vi "ConvertTemperatureToVoltage.vi"(1 "Température\nde consigne":dbl) -> (0 "Numérique":dbl)   [LabVIEW 2021]
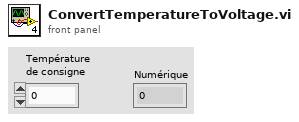
[diagram p1: front panel]
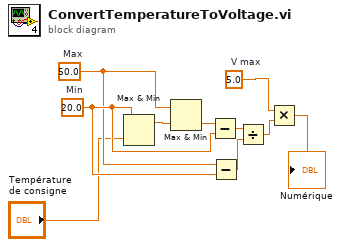
[diagram p0: block diagram]
diagram:
  w9 = 5.0  # V max
  w4 = 50.0  # Max
  w5 = 20.0  # Min
  n1 = Max & Min(x=w5, y="Température\nde consigne") -> (max(x,y)=w2:dbl)  [unwired: 1 out]
  n2 = Max & Min(x=w4, y=w2) -> (min(x,y)=w3:dbl)  [unwired: 1 out]
  n3 = Subtract(x=w3, y=w5) -> (x-y=w6:dbl)
  n4 = Subtract(x=w4, y=w5) -> (x-y=w7:dbl)
  n5 = Divide(x=w6, y=w7) -> (x/y=w8:dbl)
  n6 = Multiply(x=w9, y=w8) -> (x*y=→"Numérique":dbl)
